vi "Initialization VI.vi"(8 "error in (no error)":errorcluster, 10 "Custom XML":string, 11 "Device Item Ref in":T1 format="%.0x") -> (0 "error out":errorcluster, 3 "Device Item Ref out":T1 format="%.0x")   [LabVIEW 2014, in "UEGO Sim System Explorer.lvlib"]
uses:
  UEGO Sim System Explorer.lvlib
  <vilib>/NI Veristand/Custom Device API/Custom Device Item Ref.ctl
  <vilib>/NI Veristand/Custom Device API/Custom Device Channel.ctl
  <vilib>/NI Veristand/Custom Device API/Custom Device Channel Type.ctl
  <vilib>/NI Veristand/Custom Device API/Custom Device API.lvlib
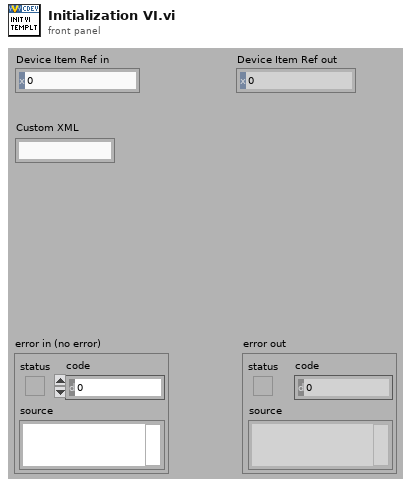
[diagram p1: front panel]
types:
  T1 = typedef "Custom Device API.lvlib/Custom Device Item Ref.ctl" = u64
  T2 = typedef "Custom Device API.lvlib/Custom Device Channel.ctl" = cluster{"Type":T3, "Units":string, "Default Value":dbl, "Faultable":bool, "Scalable":bool}
  T3 = typedef "Custom Device API.lvlib/Custom Device Channel Type.ctl" = enum16{"Input", "Output"}
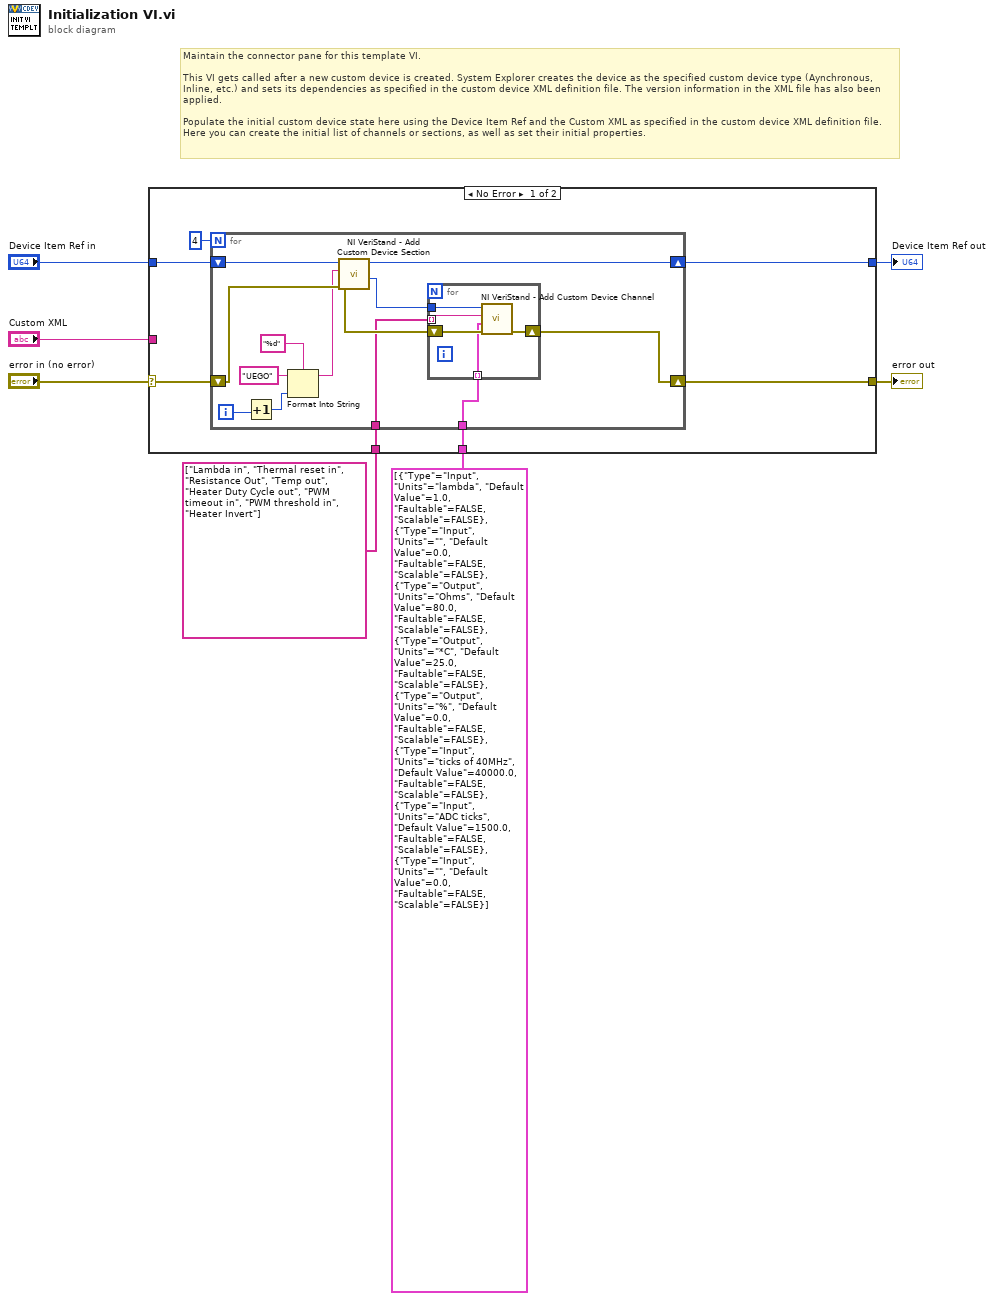
[diagram p0: block diagram]
diagram:
  # "Maintain the connector pane for this template VI.\n\nThis VI gets called after a new custom device is created. System Explorer creates the device as the specified custom device type (Aynchronous, Inline, etc.) and sets its dependencies as specified in the custom device XML definition file. The version information in the XML file has also been applied.\n\nPopulate the initial custom device state here using the Device Item Ref and the Custom XML as specified in the custom device XML definition file. Here you can create the initial list of channels or sections, as well as set their initial properties."
  n1 = case shown="No Error" "error in (no error)" {
    selector: "error in (no error)" -> [w12 w34]
    tunnel: [w11 w34] -> w7
    tunnel: [w13 w33] -> w5
    tunnel: "Device Item Ref in" -> [w14 w33]
    tunnel: "Custom XML" -> [_ _]
    tunnel: string[] ["Lambda in", "Thermal reset in", "Resistance Out", "Temp out", "Heater Duty Cycle out", "PWM timeout in", "PWM threshold in", "Heater Invert"] -> [w10 _]
    tunnel: T2[] [{"Type"=enum."Input", "Units"="lambda", "Default Value"=1.0, "Faultable"=FALSE, "Scalable"=FALSE}, {"Type"=enum."Input", "Units"="", "Default Value"=0.0, "Faultable"=FALSE, "Scalable"=FALSE}, {"Type"=enum."Output", "Units"="Ohms", "Default Value"=80.0, "Faultable"=FALSE, "Scalable"=FALSE}, {"Type"=enum."Output", "Units"="*C", "Default Value"=25.0, "Faultable"=FALSE, "Scalable"=FALSE}, {"Type"=enum."Output", "Units"="%", "Default Value"=0.0, "Faultable"=FALSE, "Scalable"=FALSE}, {"Type"=enum."Input", "Units"="ticks of 40MHz", "Default Value"=40000.0, "Faultable"=FALSE, "Scalable"=FALSE}, {"Type"=enum."Input", "Units"="ADC ticks", "Default Value"=1500.0, "Faultable"=FALSE, "Scalable"=FALSE}, {"Type"=enum."Input", "Units"="", "Default Value"=0.0, "Faultable"=FALSE, "Scalable"=FALSE}] -> [w9 _]
    frame No Error {
      n2 = for {
        N: 4 -> [_]
        shift-right: [w25] -> w13
        shift-left: w14 -> [w26]
        shift-right: [w22] -> w11
        shift-left: w12 -> [w24]
        tunnel: w10 -> [w16]
        tunnel: w9 -> [w15]
        i -> [w21]
        n3 = Increment(x=w21) -> (x+1=w20:i32)
        n4 = Format Into String(format string="%d", initial string="UEGO", w20) -> (resulting string=w17:string)  [unwired: 1 in, 1 out]
        n5 = call <vilib>:"NI VeriStand - Add Custom Device Section.vi"("error in (no error)"=w24, "Section Name"=w17, "Parent Ref in"=w26) -> ("error out"=w23:errorcluster, "Section Ptr"=w27:T1, "Parent Ref out"=w25:T1)  [unwired: 5 in, 1 out]
        n6 = for {
          tunnel: w27 -> [w32]
          shift-right: [w30] -> w22
          shift-left: w23 -> [w31]
          tunnel: w16 -> [w29] mode=indexing
          tunnel: w15 -> [w28] mode=indexing
          n7 = call <vilib>:"NI VeriStand - Add Custom Device Channel.vi"("error in (no error)"=w31, "Channel"=w28, "Channel Name"=w29, "Parent Ref in"=w32) -> ("error out"=w30:errorcluster)  [unwired: 4 in, 3 out]
        }
      }
    }
    frame Error {
    }
  }
  "error out" <- w7
  "Device Item Ref out" <- w5
